vi "UTILITY U8 Array to String.vi"(0 "U8 Data":u8[](array[numeric]), 2 "Delimiter(_)":string="_") -> (4 "String":string)   [LabVIEW 2016]
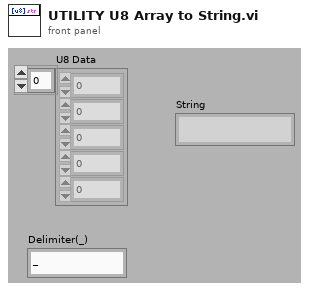
[diagram p1: front panel]
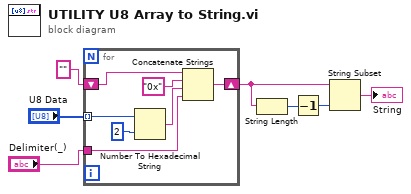
[diagram p0: block diagram]
diagram:
  n1 = for {
    tunnel: "U8 Data" -> [w14] mode=indexing
    shift-right: [w12] -> w4
    shift-left: "" -> [w10]
    tunnel: "Delimiter(_)" -> [w8]
    n2 = Number To Hexadecimal String(1:i16 2 ("width (-)"), 2:w14) -> (0:w13:string)
    n3 = Concatenate Strings(w10, "0x" ("string"), w13, w8) -> (w12:string)
  }
  n4 = String Length(string=w4) -> (length=w6:i32)
  n5 = Decrement(x=w6) -> (x-1=w5:i32)
  n6 = String Subset(string=w4, length (rest)=w5) -> (substring=→"String":string)  [unwired: 1 in]
